vi "power_supply_server_1.vi"(10 "power_supply1 load":bool, 11 "power_supply 1&2":refnum<visa-resource-name>) -> ()   [LabVIEW 2020]
uses:
  status/stop software.vi
  status/emergency stop.vi
  status/pause1.vi
  status/pause2.vi
  <instrlib>/GPD-3303/GPD-3303.lvlib
panel:
  out "pause2?":bool
  out "pause1?":bool
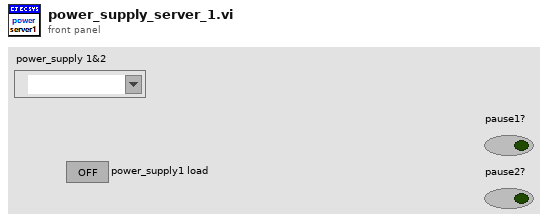
[diagram p1: front panel]
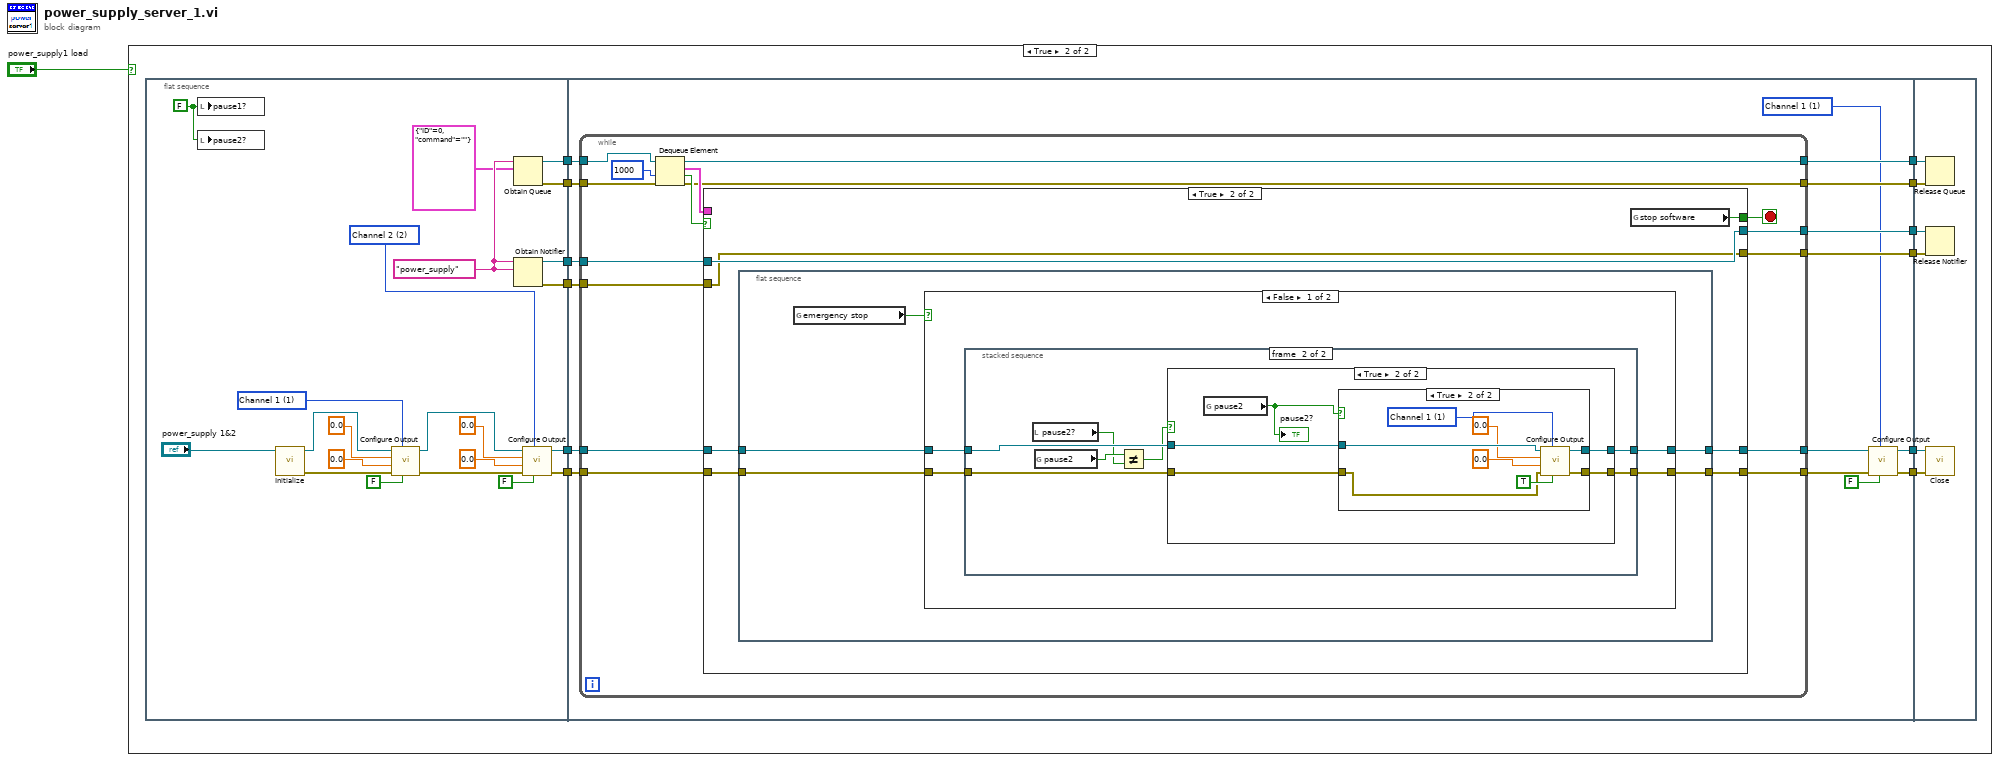
[diagram p0: block diagram]
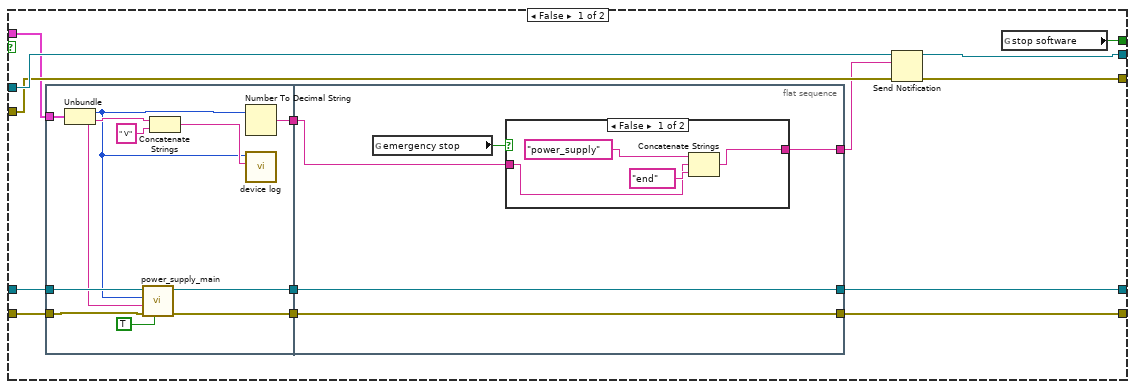
[diagram p3: hidden frame]
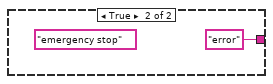
[diagram p4: hidden frame]
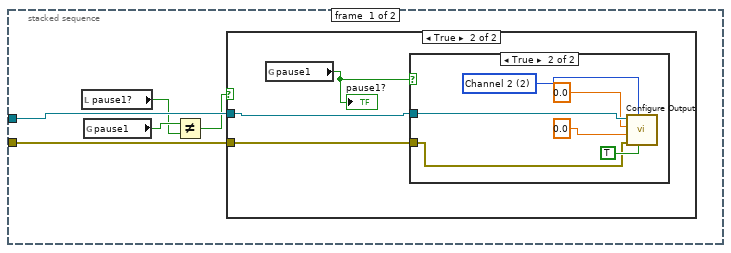
[diagram p5: hidden frame]
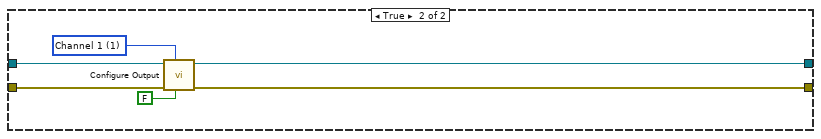
[diagram p10: hidden frame]
diagram:
  n1 = case shown="True" "power_supply1 load" {
    frame False {
    }
    frame True {
      n2 = flat-sequence {
        tunnel: [w31] -> w13
        tunnel: [w35] -> w12
        tunnel: [w34] -> w11
        tunnel: [w33] -> w10
        tunnel: [w24] -> w9
        tunnel: [w23] -> w8
        tunnel: w13 -> [w51]
        tunnel: w12 -> [w50]
        tunnel: w11 -> [w49]
        tunnel: w10 -> [w48]
        tunnel: [w47] -> w7
        tunnel: [w46] -> w6
        tunnel: [w45] -> w5
        tunnel: [w44] -> w4
        tunnel: w9 -> [w43]
        tunnel: w8 -> [w42]
        tunnel: [w37] -> w3
        tunnel: [w38] -> w2
        tunnel: w7 -> [w168]
        tunnel: w6 -> [w167]
        tunnel: w5 -> [w166]
        tunnel: w4 -> [w165]
        tunnel: w3 -> [w164]
        tunnel: w2 -> [w163]
        frame #0 {
          w14 = FALSE ("pause1?")
          w15 = 2 items=["Channel 1"=1, "Channel 2"=2] ("Channel (1: Channel 1)")
          w16 = 1 items=["Channel 1"=1, "Channel 2"=2] ("Channel (1: Channel 1)")
          w32 = "power_supply" ("name (unnamed)")
          n3 = local write "pause1?"(w14) -> ()
          n4 = local write "pause2?"(w14) -> ()
          n5 = call <instrlib>:"Initialize.vi"("VISA resource name"="power_supply 1&2") -> ("error out"=w21:errorcluster, "VISA resource name out"=w22:refnum<visa-resource-name>)  [unwired: 9 in]
          n6 = call <instrlib>:"Configure Output.vi"("Enable Output (T: Enable)"=FALSE, "Channel (1: Channel 1)"=w16, "error in (no error)"=w21, "Current Level (0.0 V)"=0.0, "Voltage Level (0.0 V)"=0.0, "VISA resource name"=w22) -> ("error out"=w25:errorcluster, "VISA resource name out"=w26:refnum<visa-resource-name>)  [unwired: 4 in]
          n7 = Obtain Queue(name (unnamed)=w32, element data type=cluster{"ID":u8, "command":string} {"ID"=0, "command"=""} ("参数")) -> (queue out=w31:refnum<queue>, error out=w35:errorcluster)  [unwired: 3 in, 1 out]
          n8 = Obtain Notifier(name (unnamed)=w32, notification data type=w32) -> (notifier out=w34:refnum<notifier>, error out=w33:errorcluster)  [unwired: 2 in, 1 out]
          n9 = call <instrlib>:"Configure Output.vi"("Enable Output (T: Enable)"=FALSE, "Channel (1: Channel 1)"=w15, "error in (no error)"=w25, "Current Level (0.0 V)"=0.0, "Voltage Level (0.0 V)"=0.0, "VISA resource name"=w26) -> ("error out"=w23:errorcluster, "VISA resource name out"=w24:refnum<visa-resource-name>)  [unwired: 4 in]
        }
        frame #1 {
          w36 = 1 items=["Channel 1"=1, "Channel 2"=2] ("Channel (1: Channel 1)")
          n10 = while {
            tunnel: w51 -> [w66]
            tunnel: w50 -> [w65]
            tunnel: w49 -> [w61]
            tunnel: w48 -> [w60]
            tunnel: [w59] -> w47
            tunnel: [w58] -> w46
            tunnel: [w57] -> w45
            tunnel: [w56] -> w44
            tunnel: w43 -> [w55]
            tunnel: w42 -> [w54]
            tunnel: [w53] -> w40
            tunnel: [w52] -> w39
            stop <- w63 stop-if-true
            n11 = Dequeue Element(queue=w66, timeout in ms (-1)=1000, error in (no error)=w65) -> (queue out=w57:refnum<queue>, element=w62:cluster{"ID":u8, "command":string}, timed out?=w64:bool, error out=w56:errorcluster)
            n12 = case shown="True" w64 {
              tunnel: [w76 w107] -> w63
              tunnel: w62 -> [w77 _]
              tunnel: w61 -> [w81 w109]
              tunnel: w60 -> [w80 w108]
              tunnel: [w79 w109] -> w59
              tunnel: [w78 w108] -> w58
              tunnel: w55 -> [w73 w106]
              tunnel: w54 -> [w72 w105]
              tunnel: [w70 w104] -> w52
              tunnel: [w69 w103] -> w53
              frame False {
                n13 = flat-sequence {
                  tunnel: w77 -> [w92]
                  tunnel: [w91] -> w75
                  tunnel: w73 -> [w88]
                  tunnel: w72 -> [w87]
                  tunnel: [w84] -> w71
                  tunnel: [w83] -> w68
                  tunnel: w75 -> [w96]
                  tunnel: [w95] -> w74
                  tunnel: w71 -> [w94]
                  tunnel: [w94] -> w70
                  tunnel: [w93] -> w69
                  tunnel: w68 -> [w93]
                  frame #0 {
                    n14 = Unbundle(w92) -> ("ID"=w85:u8, "command"=w86:string)
                    n15 = call "power_supply_main.vi"("Enable Output (T: Enable)"=TRUE, "error in (no error)"=w87, "command"=w86, "channel"=w85, "VISA resource name"=w88) -> ("error out"=w83:errorcluster, "VISA resource name out"=w84:refnum<visa-resource-name>)  [unwired: 5 in]
                    n16 = Concatenate Strings(w86, " V" ("command")) -> (w90:string)
                    n17 = Number To Decimal String(number=w85) -> (decimal integer string=w91:string)  [unwired: 1 in]
                    n18 = call "device log.vi"("new element/subarray"=w90, "worker ID"=w85) -> ()  [unwired: 10 in]
                  }
                  frame #1 {
                    n19 = global read "emergency stop.vi" "emergency stop"() -> (w97:bool)
                    n20 = case shown="False" w97 {
                      tunnel: [w99 "error" ("notification")] -> w95
                      tunnel: w96 -> [w98 _]
                      frame False {
                        n21 = Concatenate Strings("power_supply" ("string"), w98, "end" ("notification")) -> (w99:string)
                      }
                      frame True {
                        (unwired) "emergency stop" ("power_supply_1 status")
                      }
                    }
                  }
                }
                n22 = Send Notification(notification=w74, notifier=w81, error in (no error)=w80) -> (notifier out=w79:refnum<notifier>, error out=w78:errorcluster)
                n23 = global read "stop software.vi" "stop software"() -> (w76:bool)
              }
              frame True {
                n24 = flat-sequence {
                  tunnel: w106 -> [w113]
                  tunnel: w105 -> [w112]
                  tunnel: [w111] -> w104
                  tunnel: [w110] -> w103
                  frame #0 {
                    n25 = global read "emergency stop.vi" "emergency stop"() -> (w114:bool)
                    n26 = case shown="False" w114 {
                      tunnel: w113 -> [w118 w160]
                      tunnel: w112 -> [w117 w159]
                      tunnel: [w116 w158] -> w111
                      tunnel: [w115 w157] -> w110
                      frame False {
                        n27 = stacked-sequence {
                          tunnel: w118 -> [w123 w139]
                          tunnel: w117 -> [w122 w138]
                          tunnel: [_ w134] -> w116
                          tunnel: [_ w133] -> w115
                          frame #0 {
                            n28 = local read "pause1?"() -> (w119:bool)
                            n29 = global read "pause1.vi" "pause1"() -> (w120:bool)
                            n30 = Not Equal?(x=w120, y=w119) -> (x != y?=w121:bool)
                            n31 = case shown="True" w121 {
                              tunnel: w123 -> [_ w125]
                              tunnel: w122 -> [_ w124]
                              frame False {
                              }
                              frame True {
                                n32 = global read "pause1.vi" "pause1"() -> (w126:bool)
                                "pause1?" <- w126
                                n33 = case shown="True" w126 {
                                tunnel: w125 -> [_ w130]
                                tunnel: w124 -> [_ w129]
                                frame False {
                                }
                                frame True {
                                w131 = 2 items=["Channel 1"=1, "Channel 2"=2] ("Channel (1: Channel 1)")
                                n34 = call <instrlib>:"Configure Output.vi"("Enable Output (T: Enable)"=TRUE, "Channel (1: Channel 1)"=w131, "error in (no error)"=w129, "Current Level (0.0 V)"=0.0, "Voltage Level (0.0 V)"=0.0, "VISA resource name"=w130) -> ()  [unwired: 4 in, 2 out]
                                }
                                }
                              }
                            }
                          }
                          frame #1 {
                            n35 = local read "pause2?"() -> (w135:bool)
                            n36 = global read "pause2.vi" "pause2"() -> (w136:bool)
                            n37 = Not Equal?(x=w136, y=w135) -> (x != y?=w137:bool)
                            n38 = case shown="True" w137 {
                              tunnel: w139 -> [w141 w145]
                              tunnel: w138 -> [w140 w144]
                              tunnel: [w141 w143] -> w134
                              tunnel: [w140 w142] -> w133
                              frame False {
                              }
                              frame True {
                                n39 = global read "pause2.vi" "pause2"() -> (w146:bool)
                                "pause2?" <- w146
                                n40 = case shown="True" w146 {
                                tunnel: w145 -> [w148 w154]
                                tunnel: [w148 w152] -> w143
                                tunnel: w144 -> [w147 w153]
                                tunnel: [w147 w151] -> w142
                                frame False {
                                }
                                frame True {
                                w155 = 1 items=["Channel 1"=1, "Channel 2"=2] ("Channel (1: Channel 1)")
                                n41 = call <instrlib>:"Configure Output.vi"("Enable Output (T: Enable)"=TRUE, "Channel (1: Channel 1)"=w155, "error in (no error)"=w153, "Current Level (0.0 V)"=0.0, "Voltage Level (0.0 V)"=0.0, "VISA resource name"=w154) -> ("error out"=w151:errorcluster, "VISA resource name out"=w152:refnum<visa-resource-name>)  [unwired: 4 in]
                                }
                                }
                              }
                            }
                          }
                        }
                      }
                      frame True {
                        w161 = 1 items=["Channel 1"=1, "Channel 2"=2] ("Channel (1: Channel 1)")
                        n42 = call <instrlib>:"Configure Output.vi"("Enable Output (T: Enable)"=FALSE, "Channel (1: Channel 1)"=w161, "error in (no error)"=w159, "VISA resource name"=w160) -> ("error out"=w157:errorcluster, "VISA resource name out"=w158:refnum<visa-resource-name>)  [unwired: 6 in]
                      }
                    }
                  }
                }
                n43 = global read "stop software.vi" "stop software"() -> (w107:bool)
              }
            }
          }
          n44 = call <instrlib>:"Configure Output.vi"("Enable Output (T: Enable)"=FALSE, "Channel (1: Channel 1)"=w36, "error in (no error)"=w40, "VISA resource name"=w39) -> ("error out"=w38:errorcluster, "VISA resource name out"=w37:refnum<visa-resource-name>)  [unwired: 6 in]
        }
        frame #2 {
          n45 = Release Queue(queue=w166, error in (no error)=w165) -> ()  [unwired: 1 in, 3 out]
          n46 = Release Notifier(notifier=w168, error in (no error)=w167) -> ()  [unwired: 1 in, 3 out]
          n47 = call <instrlib>:"Close.vi"("error in (no error)"=w163, "VISA resource name"=w164) -> ()  [unwired: 9 in, 1 out]
        }
      }
    }
  }
